vi "Write Rx Message.vi"(8 "error in (no error)":errorcluster, 10 "Rx Message":string, 11 "RxTx in":refnum<class "CCS_RxTx.lvclass">) -> (0 "error out":errorcluster, 3 "RxTx out":refnum<class "CCS_RxTx.lvclass">)   [LabVIEW 2018, in "CCS_RxTx.lvclass"]
uses:
  CCS_RxTx.lvclass
  CCS_RxTx.lvclass/CCS_RxTx.ctl
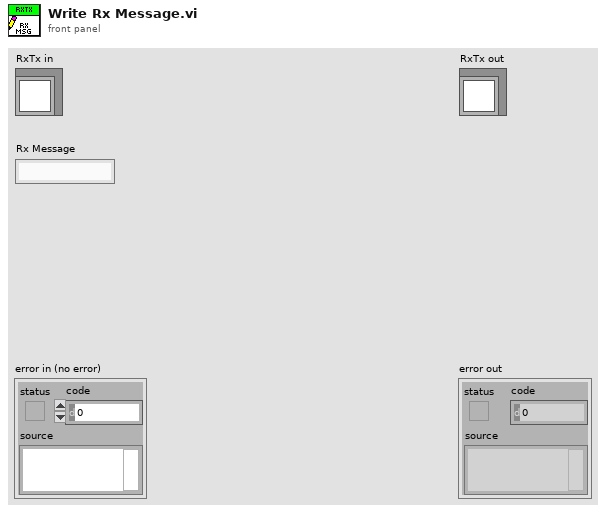
[diagram p1: front panel]
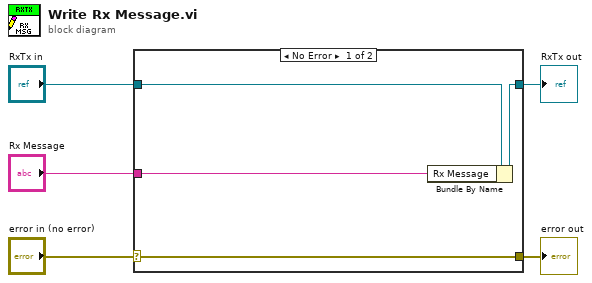
[diagram p0: block diagram]
diagram:
  n1 = case shown="No Error" "error in (no error)" {
    selector: "error in (no error)" -> [w9 w10]
    tunnel: [w9 w10] -> w4
    tunnel: [w7 w11] -> w2
    tunnel: "RxTx in" -> [w8 w11]
    tunnel: "Rx Message" -> [w6 _]
    frame No Error {
      n2 = Bundle By Name(cluster=w8, "Rx Message"=w6) -> (w7:refnum<class "CCS_RxTx.lvclass">)
    }
    frame Error {
    }
  }
  "error out" <- w4
  "RxTx out" <- w2
